vi "Populate For Index.vi"(8 "error in (no error)":errorcluster, 9 "Enum Alias":string, 10 "Enum Index":u32, 11 "Enum in":refnum<class "Enum.lvclass">) -> (0 "error out":errorcluster, 3 "Enum out":refnum<class "Enum.lvclass">)   [LabVIEW 2020, in "Data.lvlib" / "Enum.lvclass"]
uses:
  Enum.lvclass
  Enum.lvclass/Enum.ctl
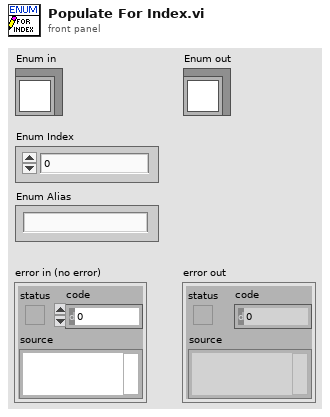
[diagram p1: front panel]
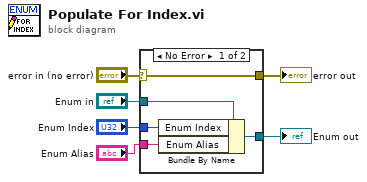
[diagram p0: block diagram]
diagram:
  n1 = case shown="No Error" "error in (no error)" {
    selector: "error in (no error)" -> [w11 w12]
    tunnel: [w11 w12] -> w5
    tunnel: [w9 w13] -> w3
    tunnel: "Enum in" -> [w10 w13]
    tunnel: "Enum Index" -> [w8 _]
    tunnel: "Enum Alias" -> [w7 _]
    frame No Error {
      n2 = Bundle By Name(cluster=w10, "Enum Index"=w8, "Enum Alias"=w7) -> (w9:refnum<class "Enum.lvclass">)
    }
    frame Error {
    }
  }
  "error out" <- w5
  "Enum out" <- w3
